vi "BCDToDecimal.vi"(11 "BCD":u8 format="%02d") -> (3 "U8":u8 format="%0d")   [LabVIEW 2019]
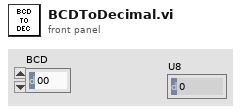
[diagram p1: front panel]
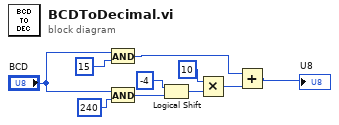
[diagram p0: block diagram]
diagram:
  n1 = And(x="BCD", y=u8 15) -> (x .and. y?=w10:u8)
  n2 = And(x="BCD", y=u8 240) -> (x .and. y?=w5:u8)
  n3 = Logical Shift(y=i16 -4, x=w5) -> (x << y=w7:u8)
  n4 = Multiply(x=u8 10, y=w7) -> (x*y=w9:u8)
  n5 = Add(x=w10, y=w9) -> (x+y=→"U8":u8)
